vi "Parse ERD Read Expected Data.vi"(0 "Read ERD List":T1[](array[typedef]) {"ERD Number" format="%.0x"}, 11 "Error In":errorcluster) -> (8 "Expected Data":string, 15 "Error Out":errorcluster)   [LabVIEW 2020, in "GEA2_Toolkit.lvlib"]
uses:
  library/GEA2_Toolkit.lvlib
  type defs/ERD Read Data In.ctl
  type defs/Data Type.ctl
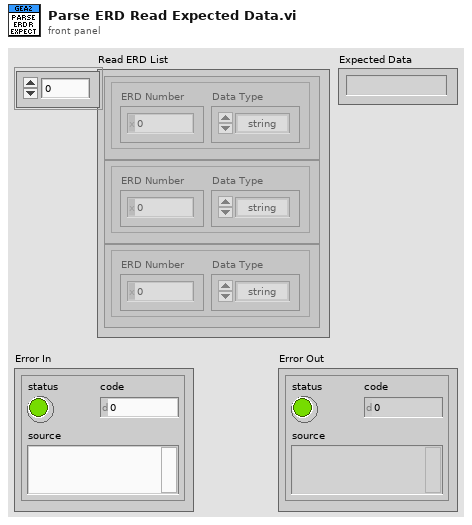
[diagram p1: front panel]
types:
  T1 = typedef "GEA2_Toolkit.lvlib/ERD Read Data In.ctl" = cluster{"ERD Number":u16, "Data Type":T2}
  T2 = typedef "GEA2_Toolkit.lvlib/Data Type.ctl" = enum16{"string", "boolean", "uint8_t", "uint16_t", "uint32_t", "uint64_t", "int8_t", "int16_t", "int32_t", "int64_t"}
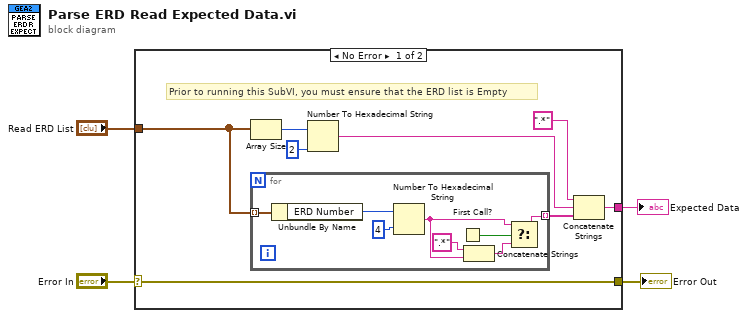
[diagram p0: block diagram]
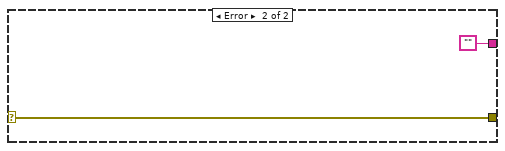
[diagram p2: hidden frame]
diagram:
  n1 = case shown="No Error" "Error In" {
    selector: "Error In" -> [w5 w22]
    tunnel: [w9 ""] -> w4
    tunnel: "Read ERD List" -> [w6 _]
    tunnel: [w5 w22] -> w2
    frame No Error {
      # "Prior to running this SubVI, you must ensure that the ERD list is Empty"
      n2 = Array Size(array=w6) -> (size(s)=w11:i32)
      n3 = for {
        tunnel: w6 -> [w20] mode=indexing
        tunnel: [w13] -> w12 mode=indexing
        n4 = Unbundle By Name(w20) -> ("ERD Number"=w19:u16)
        n5 = Number To Hexadecimal String(1:i16 4 ("width (-)"), 2:w19) -> (0:w14:string)
        n6 = First Call?() -> (First Call?: T/F=w16:bool)
        n7 = Concatenate Strings(".*" ("string"), w14) -> (w15:string)
        n8 = Select(t=w14, s=w16, f=w15) -> (s? t:f=w13:string)
      }
      n9 = Number To Hexadecimal String(1:i16 2 ("width (-)"), 2:w11) -> (0:w8:string)
      n10 = Concatenate Strings(".*" ("string"), w8, w12) -> (w9:string)
    }
    frame Error {
    }
  }
  "Expected Data" <- w4
  "Error Out" <- w2
